vi "输出调用01.vi"(0 "输出簇":cluster{"用户名":string, "项目名称":string}, 7 "数组":string[][](array[string]), 9 "字符串":string, 11 "输出簇 2":T1, 12 "Str引用句柄":refnum<vi>) -> ()   [LabVIEW 2020]
uses:
  <vilib>/numeric/Random Number (Range) DBL.vi
  <vilib>/Utility/miscctls.llb/LVDateTimeRec.ctl
panel:
  out "压力":dbl
  out "数组 6":dbl[][](array[numeric])
  out "水质":dbl
  out "温度":dbl
  out "输出 3":dbl
  out "输出 2":dbl
  out "创建的路径":path
  out "路径 2":path
  out "路径":path
  out "错误输出":errorcluster
  out "数组 5":dbl[](array[numeric])
  out "数组 4":dbl[](array[numeric])
  out "文本":string[](array[string])
  out "数组 3":dbl[](array[numeric])
  out "数组 2":dbl[](array[numeric])
  out "错误输出 2":errorcluster caption="错误输出"
  out "元素":string
  out "数值 3":i32
  out "Numeric":i32
  in  "数值":u32
  out "输出 1":dbl
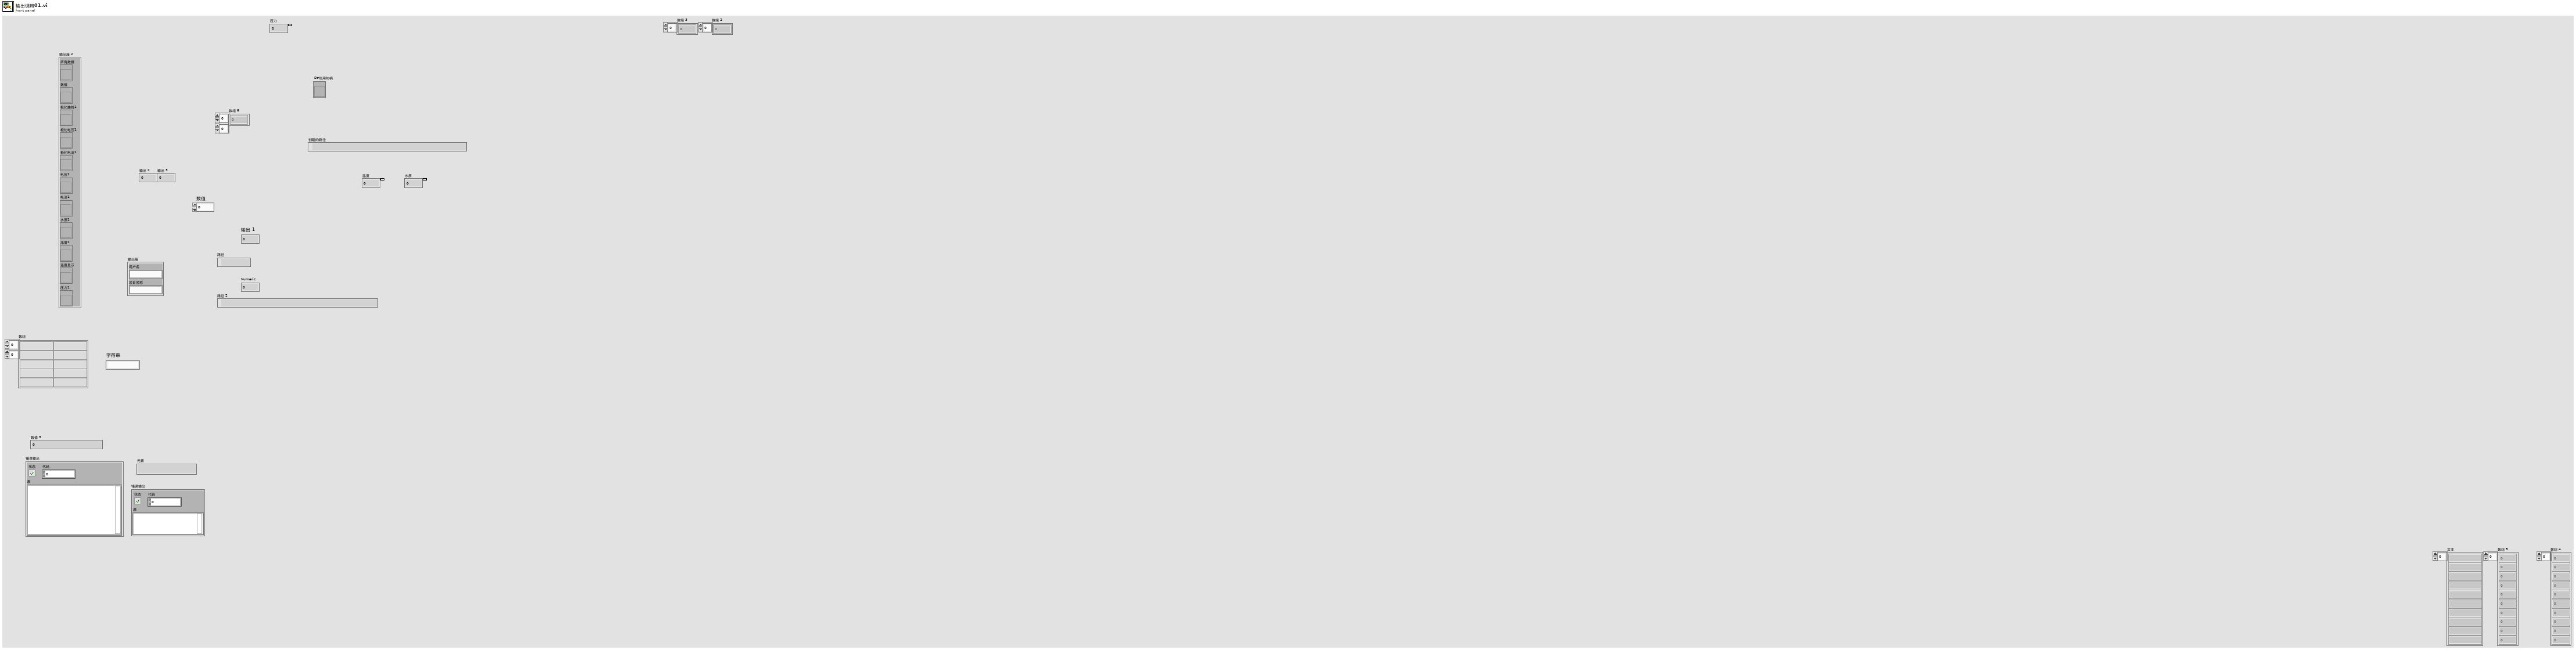
[diagram p1: front panel]
types:
  T1 = cluster{"所有数据":refnum<vi>, "数值":refnum<vi>, "极化曲线1":refnum<vi>, "极化电压1":refnum<vi>, "极化电流1":refnum<vi>, "电压1":refnum<vi>, "电流1":refnum<vi>, "水质1":refnum<vi>, "温度1":refnum<vi>, "温度显示":refnum<vi>, "压力1":refnum<vi>}
  T2 = enum16{"open", "replace", "create", "open or create", "replace or create", "replace or create with confirmation"}
  T3 = typedef "LVDateTimeRec.ctl" = cluster{"fractional second":dbl, "second":i32, "minute":i32, "hour":i32, "day of month":i32, "month":i32, "year":i32, "day of week":i32, "day of year":i32, "DST":i32}
  T4 = enum16{"open", "open or create", "create or replace", "create", "open (read-only)"}
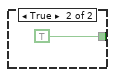
[diagram p3: hidden frame]
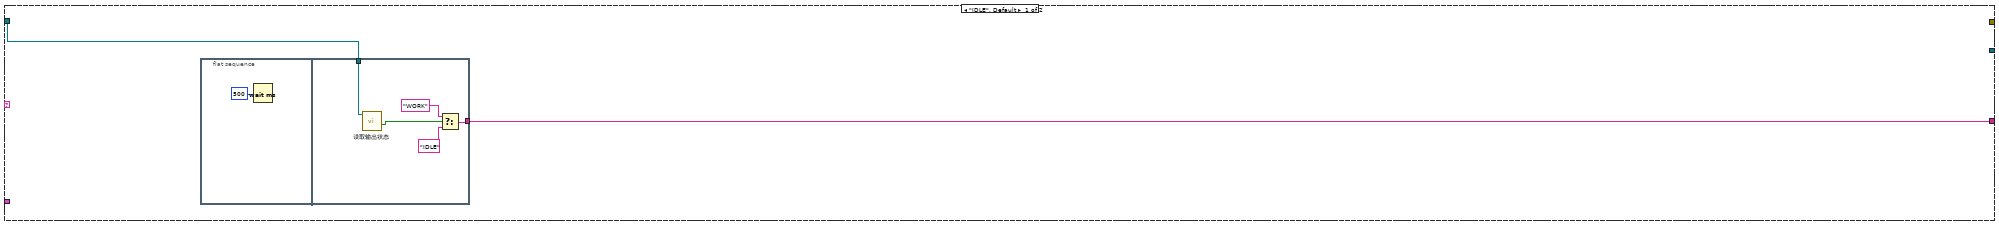
[diagram p5: hidden frame]
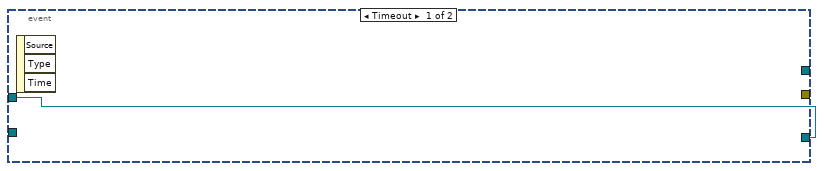
[diagram p6: hidden frame]
diagram:
  w16 = "\\" ("string")
  (unwired) dbl[] [] ("数组 4")
  n1 = Unbundle By Name("输出簇") -> ("用户名"=w13:string, "项目名称"=w12:string)
  n2 = Get Date/Time In Seconds() -> (seconds since 1Jan1904=w34:timestamp)
  n3 = Format Date/Time String(time format string (%c)="%y-%m-%d[%H-%M]", seconds (now)=w34) -> (date/time string=w15:string)  [unwired: 1 in]
  n4 = property on="输出簇 2" class="Clust (严格)"() -> ("Value"=w6:T1)  [unwired: 2 in, 2 out]
  n5 = Concatenate Strings("C:\\Users\\526computer\\Desktop", w16, "TEMPDATA\\" ("string"), w13, w16, w12, w16, "CH1\\" ("string"), w15) -> (w32:string)
  n6 = String To Path(string=w32) -> (path=w31:path)
  n7 = Create Folder(path (use dialog)=w31) -> (created path=w4:path)  [unwired: 2 in, 2 out]
  "创建的路径" <- w4
  n8 = Path To String(path=w4) -> (string=w30:string)
  n9 = Path To String(path=w4) -> (string=w2:string)
  n10 = Concatenate Strings(w30, "\\" ("string"), "通道1 索引.txt" ("string")) -> (w22:string)
  n11 = property class="Str"(reference="Str引用句柄", "Value"=w2) -> ()  [unwired: 1 in, 2 out]
  n12 = String To Path(string=w22) -> (path=w21:path)
  "路径 2" <- w21
  n13 = Unbundle By Name(w6) -> ("极化曲线1"=w11:refnum<vi>)
  n14 = property on="数组 6" class="Arr (严格)"("Value"=dbl[][] [] ("数组 6")) -> (error out=w8:errorcluster)  [unwired: 2 in, 1 out]
  n15 = Open/Create/Replace File(file path (use dialog)=w21, operation (0:open)=T2."replace or create") -> (refnum out=w20:refnum<file>)  [unwired: 4 in, 2 out]
  n16 = while {
    tunnel: w20 -> [w46]
    tunnel: [w45] -> w18
    tunnel: [w44] -> w19
    shift-right: [w42] -> _
    shift-left: w11 -> [w43]
    tunnel: w8 -> [_]
    stop <- FALSE stop-if-true
    n17 = event shown="[1] \"数值\": 值改变" {
      selector: _ -> [_ _]
      dyn-events: _ -> [_ _]
      timeout: 100 -> [_ _]
      tunnel: w46 -> [_ w64]
      tunnel: [_ w58] -> w45
      tunnel: [_ w57] -> w44
      tunnel: w43 -> [w49 w53]
      tunnel: [w49 w52] -> w42
      event Timeout {
        n18 = event-data() -> ()  [unwired: 1 in, 3 out]
      }
      event "数值": Value Change {
        n19 = event-data() -> ()  [unwired: 1 in, 6 out]
        n20 = local read "输出 3"() -> (w54:dbl)
        n21 = local read "输出 2"() -> (w55:dbl)
        n22 = property on="Numeric" class="DigNum (严格)"() -> ("Value"=w63:i32)  [unwired: 2 in, 2 out]
        n23 = Build Array(w55, w54) -> (w56:dbl[])
        n24 = Format Into String(w63) -> (resulting string=w62:string)  [unwired: 3 in, 1 out]
        n25 = property on="数组 6" class="Arr (严格)"() -> ("Value"=w51:dbl[][])  [unwired: 2 in, 2 out]
        n26 = Write to Text File(file (use dialog)=w64, text=w62) -> (refnum out=w61:refnum<file>, error out=w60:errorcluster)  [unwired: 2 in, 1 out]
        n27 = Insert Into Array(array=w51, new element=w56) -> (w50:dbl[][])  [unwired: 2 in]
        n28 = property on="数组 6" class="Arr (严格)"("Value"=w50) -> ()  [unwired: 2 in, 2 out]
        n29 = Write to Text File(file (use dialog)=w61, text="\r\n", error in=w60) -> (refnum out=w58:refnum<file>, error out=w57:errorcluster)  [unwired: 1 in, 1 out]
        n30 = property class="Arr (严格)"(reference=w53, "Value"=w50) -> (reference out=w52:refnum<vi>)  [unwired: 1 in, 1 out]
      }
    }
  }
  n31 = Path To String(path=w4) -> (string=w25:string)
  n32 = Concatenate Strings(w25, "\\" ("string"), "通道1 数据.txt" ("string")) -> (w24:string)
  n33 = String To Path(string=w24) -> (path=w23:path)
  "路径" <- w23
  n34 = Close File(refnum=w18, error in=w19) -> ()  [unwired: 2 out]
  n35 = Open/Create/Replace File(file path (use dialog)=w23, operation (0:open)=T2."replace or create" ("操作(0:open)")) -> (refnum out=w10:refnum<file>, error out=w38:errorcluster)  [unwired: 4 in, 1 out]
  n36 = disable-structure shown="禁用" {
    disable-tunnel: [w65 _] -> w41
    frame Disabled {
      n37 = flat-sequence {
        tunnel: [w89] -> w84
        tunnel: [w86] -> w83
        tunnel: w84 -> [w93]
        tunnel: [w93] -> w82
        tunnel: [w92] -> w81
        tunnel: w83 -> [w92]
        tunnel: ["字符串"] -> w80
        tunnel: w82 -> [w95]
        tunnel: w81 -> [w96]
        tunnel: [w96] -> w79
        tunnel: [w95] -> w78
        tunnel: [w94] -> w77
        tunnel: w80 -> [w94]
        tunnel: w79 -> [w103]
        tunnel: w78 -> [w104]
        tunnel: [w106] -> w76
        tunnel: [w105] -> w75
        tunnel: [w104] -> w74
        tunnel: [w103] -> w73
        tunnel: [w102] -> w65
        tunnel: w77 -> [w101]
        tunnel: w76 -> [w119]
        tunnel: w75 -> [w118]
        tunnel: [w115] -> w72
        tunnel: w74 -> [w115]
        tunnel: [w114] -> w71
        tunnel: w73 -> [w114]
        tunnel: [w109] -> w70
        tunnel: [w108] -> w69
        tunnel: ["输出簇 2"] -> w68
        tunnel: w72 -> [w148]
        tunnel: w71 -> [w152]
        tunnel: w70 -> [w151]
        tunnel: w69 -> [w150]
        tunnel: [w149] -> w67
        tunnel: [w145] -> w66
        tunnel: w68 -> [w144]
        tunnel: w67 -> [w205]
        tunnel: w66 -> [w203]
        frame #0 {
          n38 = property on="数值" class="DigNum (严格)"("Value"=i64 0 ("数值")) -> ()  [unwired: 2 in, 2 out]
          n39 = Index Array(array="数组", index (col)=5 ("禁用的索引 (列)")) -> (element=w86:string[])  [unwired: 1 in]
          n40 = Index Array(array="数组", index (col)=3 ("禁用的索引 (列)")) -> (element=w89:string[])  [unwired: 1 in]
        }
        frame #1 {
          n41 = VISA Close(VISA resource name="字符串") -> ()  [unwired: 1 in, 1 out]
        }
        frame #2 {
        }
        frame #3 {
          n42 = VISA Open(VISA resource name=w101) -> (VISA resource name=w102:refnum<visa-resource-name>, error out=w99:errorcluster)  [unwired: 4 in]
          n43 = call "remote.vi"("error in (no error)"=w99, "VISA resource name"=w102) -> ("error out"=w97:errorcluster, "VISA resource name out"=w98:refnum<visa-resource-name>)  [unwired: 8 in]
          n44 = call "enableoutput.vi"("error in (no error)"=w97, "Enable OutPut(True)"=FALSE, "VISA resource name"=w98) -> ("error out"=w105:errorcluster, "VISA resource name out"=w106:refnum<visa-resource-name>)  [unwired: 7 in]
        }
        frame #4 {
          n45 = flat-sequence {
            tunnel: w119 -> [w124]
            tunnel: w118 -> [w123]
            tunnel: [w121] -> w117
            tunnel: [w120] -> w116
            tunnel: w117 -> [w130]
            tunnel: w116 -> [w129]
            tunnel: [w126] -> w113
            tunnel: [w125] -> w112
            tunnel: w113 -> [w136]
            tunnel: w112 -> [w135]
            tunnel: [w133] -> w111
            tunnel: [w132] -> w110
            tunnel: w111 -> [w142]
            tunnel: w110 -> [w141]
            tunnel: [w138] -> w109
            tunnel: [w137] -> w108
            frame #0 {
              n46 = call "priority.vi"("error in (no error)"=w123, "字符串"="CURR", "VISA resource name"=w124) -> ("error out"=w120:errorcluster, "VISA resource name out"=w121:refnum<visa-resource-name>)  [unwired: 7 in]
            }
            frame #1 {
              n47 = call "初始化电压电流.vi"("error in (no error)"=w129, "输入 2"=0.1, "输入 1"=15.0, "VISA resource name"=w130) -> ("error out"=w125:errorcluster, "VISA resource name out"=w126:refnum<visa-resource-name>)  [unwired: 6 in]
            }
            frame #2 {
              n48 = call "限制电流.vi"("error in (no error)"=w135, "OCP Delay(0)"=3.0, "数值"=120.0 ("OCP Level(0)"), "VISA resource name"=w136) -> ("error out"=w132:errorcluster, "VISA resource name out"=w133:refnum<visa-resource-name>)  [unwired: 6 in]
            }
            frame #3 {
              n49 = call "限制电压.vi"("error in (no error)"=w141, "OVP Delay(0)"=3.0, "OVP Level(0)"=20.0, "VISA resource name"=w142) -> ("error out"=w137:errorcluster, "VISA resource name out"=w138:refnum<visa-resource-name>)  [unwired: 6 in]
            }
          }
        }
        frame #5 {
          n50 = Unbundle By Name(w144) -> ("数值"=w143:refnum<vi>)
          n51 = Search 1D Array(1D array=w148, element=" " ("元素")) -> (index of element=w146:i32)  [unwired: 1 in]
          n52 = for {
            N: w146 -> [_]
            tunnel: w152 -> [w174] mode=indexing
            tunnel: w148 -> [w171] mode=indexing
            tunnel: w150 -> [w169]
            shift-right: [w164] -> w149
            shift-left: w151 -> [w170]
            tunnel: [w161] -> w145
            shift-right: [w155] -> _
            shift-left: w143 -> [w156]
            i -> [w154]
            n53 = Scan From String(input string=w174) -> (output 1=w173:dbl)  [unwired: 4 in, 3 out]
            n54 = Scan From String(input string=w171) -> (output 1=w168:dbl)  [unwired: 4 in, 3 out]
            "输出 1" <- w168
            n55 = Multiply(x=w173, y=1000.0) -> (x*y=w165:dbl)
            n56 = flat-sequence {
              tunnel: w170 -> [w179]
              tunnel: w169 -> [w178]
              tunnel: w168 -> [w177]
              tunnel: [w176] -> w167
              tunnel: [w175] -> w166
              tunnel: w167 -> [w182]
              tunnel: w166 -> [w183]
              tunnel: [w181] -> w163
              tunnel: [w180] -> w162
              tunnel: w165 -> [w193]
              tunnel: w163 -> [w192]
              tunnel: [w192] -> w160
              tunnel: [w191] -> w158
              tunnel: w162 -> [w191]
              tunnel: w160 -> [w198]
              tunnel: [w198] -> w159
              tunnel: w158 -> [w197]
              tunnel: [w197] -> w157
              tunnel: w156 -> [w196]
              tunnel: [w195] -> w155
              tunnel: w153 -> [w194]
              tunnel: [w201] -> w164
              tunnel: w159 -> [w202]
              tunnel: w157 -> [w200]
              tunnel: [w199] -> w161
              frame #0 {
                n57 = call "设置电流.vi"("error in (no error)"=w178, "输入 1"=w177, "VISA resource name"=w179) -> ("error out"=w175:errorcluster, "VISA resource name out"=w176:refnum<visa-resource-name>)  [unwired: 7 in]
              }
              frame #1 {
                n58 = First Call?() -> (First Call?: T/F=w184:bool)
                n59 = case shown="真" w184 {
                  tunnel: w182 -> [w185 w190]
                  tunnel: w183 -> [_ w189]
                  tunnel: [w185 w187] -> w181
                  tunnel: [_ w186] -> w180
                  frame False {
                  }
                  frame True {
                    n60 = call "enableoutput.vi"("error in (no error)"=w189, "Enable OutPut(True)"=TRUE, "VISA resource name"=w190) -> ("error out"=w186:errorcluster, "VISA resource name out"=w187:refnum<visa-resource-name>)  [unwired: 7 in]
                  }
                }
              }
              frame #2 {
                n61 = Wait (ms)(milliseconds to wait=w193) -> ()  [unwired: 1 out]
              }
              frame #3 {
                n62 = property on="数值" class="DigNum (严格)"("Val(Sgnl)"=w194) -> ()  [unwired: 2 in, 2 out]
                n63 = property class="DigNum (严格)"(reference=w196, "Val(Sgnl)"=w194) -> (reference out=w195:refnum<vi>)  [unwired: 1 in, 1 out]
              }
              frame #4 {
                n64 = call "remote.vi"("error in (no error)"=w200, "VISA resource name"=w202) -> ("error out"=w199:errorcluster, "VISA resource name out"=w201:refnum<visa-resource-name>)  [unwired: 8 in]
              }
            }
            n65 = Increment(x=w154) -> (x+1=w153:i32)
          }
        }
        frame #6 {
          n66 = flat-sequence {
            tunnel: w205 -> [w209]
            tunnel: [w208] -> w204
            tunnel: w203 -> [w206]
            tunnel: w204 -> [w210]
            frame #0 {
              n67 = call "enableoutput.vi"("error in (no error)"=w206, "Enable OutPut(True)"=FALSE, "VISA resource name"=w209) -> ("VISA resource name out"=w208:refnum<visa-resource-name>)  [unwired: 7 in, 1 out]
            }
            frame #1 {
              n68 = VISA Close(VISA resource name=w210) -> ()  [unwired: 1 in, 1 out]
            }
            frame #2 {
              n69 = flat-sequence {
                tunnel: [w230] -> w223
                tunnel: [w229] -> w222
                tunnel: [w228] -> w221
                tunnel: [w227] -> w220
                tunnel: [w226] -> w219
                tunnel: [w224] -> w212
                tunnel: w223 -> [w279]
                tunnel: w222 -> [w278]
                tunnel: [w296] -> w213
                tunnel: [w295] -> w214
                tunnel: w221 -> [w291]
                tunnel: [w290] -> w215
                tunnel: w220 -> [w282]
                tunnel: w219 -> [w283]
                tunnel: [w280] -> w216
                tunnel: [w281] -> w217
                tunnel: [w280] -> w218
                tunnel: w212 -> [w274]
                tunnel: [w273] -> w211
                tunnel: w218 -> [w354]
                tunnel: w217 -> [w353]
                tunnel: w216 -> [w372]
                tunnel: w215 -> [w378]
                tunnel: w214 -> [w386]
                tunnel: w213 -> [w385]
                tunnel: w211 -> [w303]
                frame #0 {
                  n70 = property on="路径" class="Path"() -> ("Value"=w225:path)  [unwired: 2 in, 2 out]
                  n71 = Open/Create/Replace File(file path (use dialog)=w225, operation (0:open)=T2."open" ("操作(0:open)")) -> (refnum out=w233:refnum<file>, error out=w232:errorcluster)  [unwired: 4 in, 1 out]
                  n72 = while {
                    tunnel: w233 -> [w270]
                    tunnel: w232 -> [w268]
                    tunnel: [w267] -> w231
                    tunnel: [w241] -> w230 mode=indexing
                    tunnel: [w240] -> w229 mode=indexing
                    tunnel: [w256] -> _
                    tunnel: [w244] -> w228 mode=indexing
                    tunnel: [w239] -> w227 mode=indexing
                    tunnel: [w238] -> w226 mode=indexing
                    tunnel: [w235] -> w224 mode=indexing
                    i -> [w237]
                    stop <- w257 stop-if-true
                    n73 = Read from Text File(file (use dialog)=w270, count=1 ("计数"), error in=w268) -> (refnum out=w267:refnum<file>, text=w261:string[], error out=w256:errorcluster)  [unwired: 1 in, 1 out]
                    n74 = Unbundle By Name(w256) -> ("status"=w264:bool, "code"=w266:i32)
                    n75 = Equal?(x=w266, y=4) -> (x = y?=w263:bool)
                    n76 = Index Array(array=w261, index=0 ("索引")) -> (element=w258:string)
                    "元素" <- w258
                    n77 = And(x=w264, y=w263) -> (x .and. y?=w262:bool)
                    n78 = case shown="假" w262 {
                      tunnel: [FALSE TRUE] -> w257
                      frame False {
                      }
                      frame True {
                      }
                    }
                    n79 = Search/Split String(string=w258, search string/char (-)="电流：" ("正则表达式")) -> (substring before match=w253:string, match + rest of string=w243:string)  [unwired: 1 in, 1 out]
                    n80 = Scan From String(format string="%d-%d-%d %d:%d:%d" ("格式字符串"), input string=w253) -> (error out=→"错误输出 2":errorcluster, output 1=w252:i32, output 2=w251:i32, output 3=w250:i32, output 4=w249:i32, output 5=w248:i32, output 6=w247:i32)  [unwired: 8 in, 2 out]
                    n81 = Bundle By Name(cluster=T3 {"fractional second"=0.9035696983337402, "second"=34, "minute"=35, "hour"=15, "day of month"=21, "month"=2, "year"=2022, "day of week"=2, "day of year"=52, "DST"=0} ("日期时间记录"), "second"=w247, "minute"=w248, "hour"=w249, "day of month"=w250, "month"=w251, "year"=w252) -> (w245:T3)
                    n82 = Scan From String(format string="电流：%f 电压：%f 温度：%f 水质：%f 压力：%f" ("格式字符串"), input string=w243) -> (error out=w236:errorcluster, output 1=w241:dbl, output 2=w240:dbl, output 3=w239:dbl, output 4=w238:dbl, output 5=w235:dbl)  [unwired: 7 in, 2 out]
                    n83 = call <vilib>:"Clear Errors.vi"("error in (no error)"=w236) -> ()  [unwired: 5 in, 2 out]
                    n84 = Date/Time To Seconds(2:w245) -> (0:w244:timestamp)  [unwired: 1 in]
                    "数值 3" <- w237
                  }
                  n85 = Close File(refnum=w231) -> ()  [unwired: 1 in, 2 out]
                }
                frame #1 {
                  n86 = Array Size(array=w278) -> (size(s)=w298:i32)
                  n87 = Array Size(array=w279) -> (size(s)=w301:i32)
                  n88 = Array Size(array=w291) -> (size(s)=w293:i32)
                  n89 = Array Size(array=w274) -> (size(s)=w275:i32)
                  n90 = Decrement(x=w298) -> (x-1=w299:i32)
                  n91 = Decrement(x=w301) -> (x-1=w300:i32)
                  n92 = Decrement(x=w293) -> (x-1=w294:i32)
                  n93 = Array Size(array=w282) -> (size(s)=w289:i32)
                  n94 = Array Size(array=w283) -> (size(s)=w288:i32)
                  n95 = Decrement(x=w275) -> (x-1=w277:i32)
                  n96 = Decrement(x=w289) -> (x-1=w287:i32)
                  n97 = Decrement(x=w288) -> (x-1=w284:i32)
                  n98 = Delete From Array(array=w274, length=1 ("长度"), index=w277) -> (array with subset deleted=w273:dbl[])  [unwired: 1 out]
                  n99 = Delete From Array(array=w282, length=1 ("长度"), index=w287) -> (array with subset deleted=w280:dbl[])  [unwired: 1 out]
                  n100 = Delete From Array(array=w278, length=1 ("长度"), index=w299) -> (array with subset deleted=w295:dbl[])  [unwired: 1 out]
                  n101 = Delete From Array(array=w279, length=1 ("长度"), index=w300) -> (array with subset deleted=w296:dbl[])  [unwired: 1 out]
                  n102 = Delete From Array(array=w291, length=1 ("长度"), index=w294) -> (array with subset deleted=w290:timestamp[])  [unwired: 1 out]
                  n103 = Delete From Array(array=w283, length=1 ("长度"), index=w284) -> (array with subset deleted=w281:dbl[])  [unwired: 1 out]
                  "数组 3" <- w279
                  "数组 2" <- w278
                }
                frame #2 {
                  w340 = "极化" ("组名称输入（无标题）")
                  w319 = "数据" ("组名称")
                  n104 = property on="创建的路径" class="Path"() -> ("Value"=w322:path)  [unwired: 2 in, 2 out]
                  n105 = Array Max & Min(array=w303) -> (max value=w305:dbl, max index (indices)=w307:i32, min value=w306:dbl, min index (indices)=w308:i32)
                  n106 = Array Max & Min(array=w372) -> (max value=w347:dbl, max index (indices)=w345:i32, min value=w346:dbl, min index (indices)=w344:i32)
                  n107 = Array Max & Min(array=w353) -> (max value=w351:dbl, max index (indices)=w349:i32, min value=w350:dbl, min index (indices)=w348:i32)
                  n108 = Array Size(array=w378) -> (size(s)=w377:i32)
                  n109 = Array Max & Min(array=w386) -> (max value=w399:dbl, max index (indices)=w394:i32, min value=w398:dbl, min index (indices)=w393:i32)
                  n110 = Array Max & Min(array=w385) -> (max value=w401:dbl, max index (indices)=w395:i32, min value=w402:dbl, min index (indices)=w396:i32)
                  n111 = Index Array(array=w378, index=0 ("索引")) -> (element=w375:timestamp)
                  n112 = Build Array(w306, w305, w307, w308) -> (w304:dbl[])
                  n113 = Build Array(w351, w350, w349, w348) -> (w362:dbl[])
                  n114 = Build Array(w347, w346, w345, w344) -> (w363:dbl[])
                  n115 = Decrement(x=w377) -> (x-1=w376:i32)
                  n116 = Build Array(w398, w399, w394, w393) -> (w397:dbl[])
                  n117 = Build Array(w402, w401, w396, w395) -> (w400:dbl[])
                  n118 = Path To String(path=w322) -> (string=w323:string)
                  n119 = Index Array(array=w378, index=w376) -> (element=w374:timestamp)
                  n120 = Get Date/Time In Seconds() -> (seconds since 1Jan1904=w418:timestamp)
                  n121 = Format Date/Time String(time format string (%c)="%Y-%m-%d-%H-%M-%S" ("时间格式字符串(%c)"), seconds (now)=w418) -> (date/time string=w325:string)  [unwired: 1 in]
                  n122 = Concatenate Strings(w323, "\\" ("字符串"), w325, ".tdms" ("字符串")) -> (w419:string)
                  n123 = String To Path(string=w419) -> (path=w420:path)
                  n124 = Build Array(w375, w374) -> (w373:timestamp[])
                  n125 = TDMS Open(5:FALSE ("创建索引文件？(T)"), 10:T4."create or replace" ("操作(0:open)"), 11:w420) -> (0:w331:errorcluster, 3:w333:refnum<k34>)  [unwired: 4 in]
                  n126 = Build Array("电解水实验" ("组名称"), "孙成，王彪" ("组名称"), w325, "极化曲线" ("组名称")) -> (w324:string[])
                  n127 = TDMS Set Properties(5:w324, 7:string[] ["Title", "Author", "Date/Time", "type"] ("属性名称"), 8:w331, 11:w333) -> (0:w330:errorcluster, 3:w332:refnum<k34>)  [unwired: 2 in, 2 out]
                  n128 = TDMS Set Properties(5:w373, 7:string[] ["最小值", "最大值"] ("属性名称"), 8:w330, 9:"测试时间" ("通道名称"), 10:w319, 11:w332) -> (0:w409:errorcluster, 3:w410:refnum<k34>)  [unwired: 2 out]
                  n129 = TDMS Set Properties(5:w400, 7:string[] ["最小值", "最大值", "最小索引", "最大索引"] ("属性名称"), 8:w409, 9:"电流" ("通道名称"), 10:w319, 11:w410) -> (0:w403:errorcluster, 3:w406:refnum<k34>)  [unwired: 2 out]
                  n130 = TDMS Set Properties(5:w397, 7:string[] ["最小值", "最大值", "最小索引", "最大索引"] ("属性名称"), 8:w403, 9:"电压" ("通道名称"), 10:w319, 11:w406) -> (0:w366:errorcluster, 3:w367:refnum<k34>)  [unwired: 2 out]
                  n131 = TDMS Set Properties(5:w363, 7:string[] ["最小值", "最大值", "最小索引", "最大索引"] ("属性名称"), 8:w366, 9:"温度" ("通道名称"), 10:w319, 11:w367) -> (0:w364:errorcluster, 3:w365:refnum<k34>)  [unwired: 2 out]
                  n132 = TDMS Set Properties(5:w362, 7:string[] ["最小值", "最大值", "最小索引", "最大索引"] ("属性名称"), 8:w364, 9:"水质" ("通道名称"), 10:w319, 11:w365) -> (0:w316:errorcluster, 3:w318:refnum<k34>)  [unwired: 2 out]
                  n133 = TDMS Set Properties(5:w304, 7:string[] ["最小值", "最大值", "最小索引", "最大索引"] ("属性名称"), 8:w316, 9:"压力" ("通道名称"), 10:w319, 11:w318) -> (0:w315:errorcluster, 3:w317:refnum<k34>)  [unwired: 2 out]
                  n134 = TDMS Write(0:w317, 5:"数据" ("组名称输入（无标题）"), 7:string[] ["电流"] ("通道名输入（无标题）"), 9:w385, 11:w315) -> (4:w389:refnum<k34>, 15:w388:errorcluster)  [unwired: 1 in, 2 out]
                  n135 = TDMS Write(0:w389, 5:"数据" ("组名称输入（无标题）"), 7:string[] ["电压"] ("通道名输入（无标题）"), 9:w386, 11:w388) -> (4:w381:refnum<k34>, 15:w380:errorcluster)  [unwired: 1 in, 2 out]
                  n136 = TDMS Write(0:w381, 5:"数据" ("组名称输入（无标题）"), 7:string[] ["测试时间"] ("通道名输入（无标题）"), 9:w378, 11:w380) -> (4:w356:refnum<k34>, 15:w355:errorcluster)  [unwired: 1 in, 2 out]
                  n137 = flat-sequence {
                    tunnel: [w422] -> w343
                    tunnel: w343 -> [w429]
                    tunnel: [w428] -> w335
                    tunnel: [w427] -> w334
                    frame #0 {
                      n138 = property on="路径 2" class="Path"() -> ("Value"=w421:path)  [unwired: 2 in, 2 out]
                      n139 = Open/Create/Replace File(file path (use dialog)=w421, operation (0:open)=T2."open" ("操作(0:open)")) -> (refnum out=w426:refnum<file>)  [unwired: 4 in, 2 out]
                      n140 = Read from Text File(file (use dialog)=w426, count=-1 ("计数")) -> (refnum out=w423:refnum<file>, text=w422:string[])  [unwired: 2 in, 2 out]
                      "文本" <- w422
                      n141 = Close File(refnum=w423) -> ()  [unwired: 1 in, 2 out]
                    }
                    frame #1 {
                      n142 = for {
                        tunnel: w429 -> [w438] mode=indexing
                        tunnel: [w436] -> w428 mode=indexing
                        tunnel: [w435] -> w427 mode=indexing
                        n143 = Scan From String(format string="%d" ("格式字符串"), input string=w438) -> (output 1=w434:i32)  [unwired: 3 in, 3 out]
                        n144 = property on="数组 3" class="Arr (严格)"() -> ("Value"=w430:dbl[])  [unwired: 2 in, 2 out]
                        n145 = Decrement(x=w434) -> (x-1=w433:i32)
                        n146 = Decrement(x=w434) -> (x-1=w432:i32)
                        n147 = Index Array(array=w430, index=w433) -> (element=w436:dbl)
                        n148 = property on="数组 2" class="Arr (严格)"() -> ("Value"=w431:dbl[])  [unwired: 2 in, 2 out]
                        n149 = Index Array(array=w431, index=w432) -> (element=w435:dbl)
                      }
                      "数组 5" <- w428
                      "数组 4" <- w427
                    }
                  }
                  n150 = TDMS Write(0:w356, 5:"数据" ("组名称输入（无标题）"), 7:string[] ["温度"] ("通道名输入（无标题）"), 9:w354, 11:w355) -> (4:w352:refnum<k34>, 15:w361:errorcluster)  [unwired: 1 in, 2 out]
                  n151 = TDMS Write(0:w352, 5:"数据" ("组名称输入（无标题）"), 7:string[] ["水质"] ("通道名输入（无标题）"), 9:w353, 11:w361) -> (4:w312:refnum<k34>, 15:w310:errorcluster)  [unwired: 1 in, 2 out]
                  n152 = TDMS Write(0:w312, 5:"数据" ("组名称输入（无标题）"), 7:string[] ["压力"] ("通道名输入（无标题）"), 9:w303, 11:w310) -> (4:w311:refnum<k34>, 15:w309:errorcluster)  [unwired: 1 in, 2 out]
                  n153 = TDMS Write(0:w311, 5:w340, 7:string[] ["电流"] ("通道名输入（无标题）"), 9:w335, 11:w309) -> (4:w342:refnum<k34>, 15:w341:errorcluster)  [unwired: 1 in, 2 out]
                  n154 = TDMS Write(0:w342, 5:w340, 7:string[] ["电压"] ("通道名输入（无标题）"), 9:w334, 11:w341) -> (4:w337:refnum<k34>, 15:w336:errorcluster)  [unwired: 1 in, 2 out]
                  n155 = TDMS Close(8:w336, 11:w337) -> (0:→"错误输出":errorcluster)  [unwired: 1 out]
                }
              }
            }
            frame #3 {
              n156 = Request Deallocation(TRUE ("标志")) -> ()
            }
            frame #4 {
              n157 = Stop(stop? (T)=TRUE ("停止？(T)")) -> ()
            }
          }
        }
      }
    }
    frame Enabled {
    }
  }
  n158 = property on="输出簇 2" class="Clust (严格)"() -> ("Value"=w7:T1)  [unwired: 2 in, 2 out]
  n159 = while {
    shift-right: [w444] -> _
    shift-left: "IDLE" -> [w450]
    tunnel: w41 -> [w449]
    tunnel: w10 -> [w448]
    tunnel: w38 -> [w447]
    tunnel: [w446] -> w37
    tunnel: [w445] -> w36
    tunnel: w7 -> [w441]
    i -> [w443]
    stop <- FALSE stop-if-true
    n160 = Wait (ms)(milliseconds to wait=u32 500 ("等待时间（毫秒）")) -> ()  [unwired: 1 out]
    n161 = case shown="\"WORK\"" w450 {
      tunnel: [w453 w506] -> w444
      tunnel: w449 -> [w452 w514]
      tunnel: w448 -> [_ w513]
      tunnel: w447 -> [_ w511]
      tunnel: [_ w508] -> w446
      tunnel: [_ w507] -> w445
      tunnel: w441 -> [_ w493]
      frame "IDLE", Default {
        n162 = flat-sequence {
          tunnel: [w456] -> w453
          tunnel: w452 -> [w455]
          frame #0 {
            n163 = Wait (ms)(milliseconds to wait=u32 500 ("等待时间（毫秒）")) -> ()  [unwired: 1 out]
          }
          frame #1 {
            n164 = call "读取输出状态.vi"("VISA resource name"=w455) -> ("x = y?"=w459:bool)  [unwired: 7 in, 3 out]
            n165 = Select(t="WORK", s=w459, f="IDLE") -> (s? t:f=w456:string)
          }
        }
      }
      frame "WORK" {
        n166 = Unbundle By Name(w493) -> ("所有数据"=w471:refnum<vi>, "极化电压1"=w469:refnum<vi>, "极化电流1"=w492:refnum<vi>, "电压1"=w491:refnum<vi>, "电流1"=w490:refnum<vi>, "水质1"=w470:refnum<vi>, "温度1"=w468:refnum<vi>, "压力1"=w463:refnum<vi>)  [unwired: 3 out]
        n167 = flat-sequence {
          tunnel: [w526] -> w517
          tunnel: [w525] -> w516
          tunnel: w514 -> [w524]
          tunnel: w513 -> [w522]
          tunnel: [w523] -> w512
          tunnel: w511 -> [w523]
          tunnel: [w522] -> w510
          tunnel: [w518] -> w509
          tunnel: w492 -> [w521]
          tunnel: [w518] -> w486
          tunnel: [w518] -> w460
          tunnel: w517 -> [w538]
          tunnel: w516 -> [w537]
          tunnel: [w535] -> w505
          tunnel: [w534] -> w503
          tunnel: w512 -> [w532]
          tunnel: w510 -> [w533]
          tunnel: [w533] -> w501
          tunnel: [w532] -> w499
          tunnel: [w531] -> w497
          tunnel: w509 -> [w531]
          tunnel: [w528] -> w495
          tunnel: [w528] -> w489
          tunnel: [w530] -> w487
          tunnel: w486 -> [w530]
          tunnel: [w528] -> w484
          tunnel: w469 -> [w529]
          tunnel: w460 -> [w528]
          tunnel: w505 -> [w555]
          tunnel: [w555] -> w504
          tunnel: w503 -> [w554]
          tunnel: [w554] -> w502
          tunnel: w501 -> [w553]
          tunnel: [w553] -> w500
          tunnel: w499 -> [w552]
          tunnel: [w552] -> w498
          tunnel: w497 -> [w551]
          tunnel: [w551] -> w496
          tunnel: w495 -> [w550]
          tunnel: [w550] -> w494
          tunnel: w491 -> [w549]
          tunnel: w490 -> [w541]
          tunnel: w489 -> [w546]
          tunnel: [w540] -> w488
          tunnel: w487 -> [w540]
          tunnel: [w539] -> w485
          tunnel: w484 -> [w539]
          tunnel: [w643] -> w483
          tunnel: w504 -> [w643]
          tunnel: w502 -> [w626]
          tunnel: w500 -> [w630]
          tunnel: w498 -> [w629]
          tunnel: w496 -> [w628]
          tunnel: w494 -> [w616]
          tunnel: [w627] -> w481
          tunnel: [w626] -> w479
          tunnel: [w625] -> w507
          tunnel: [w612] -> w477
          tunnel: w488 -> [w612]
          tunnel: [w611] -> w475
          tunnel: w485 -> [w611]
          tunnel: [w604] -> w473
          tunnel: w470 -> [w603]
          tunnel: w468 -> [w584]
          tunnel: [w583] -> w466
          tunnel: [w582] -> w464
          tunnel: w463 -> [w568]
          tunnel: [w567] -> w461
          tunnel: w483 -> [w652]
          tunnel: [w652] -> w482
          tunnel: w481 -> [w651]
          tunnel: [w651] -> w480
          tunnel: w479 -> [w650]
          tunnel: [w650] -> w478
          tunnel: w477 -> [w649]
          tunnel: [w649] -> w476
          tunnel: w475 -> [w648]
          tunnel: [w648] -> w474
          tunnel: w473 -> [w647]
          tunnel: [w647] -> w472
          tunnel: [w646] -> w467
          tunnel: w466 -> [w646]
          tunnel: [w645] -> w465
          tunnel: w464 -> [w645]
          tunnel: [w644] -> w462
          tunnel: w461 -> [w644]
          tunnel: [w674] -> w515
          tunnel: w482 -> [w674]
          tunnel: w480 -> [w673]
          tunnel: w478 -> [w672]
          tunnel: [w671] -> w508
          tunnel: w476 -> [w666]
          tunnel: w474 -> [w663]
          tunnel: w472 -> [w657]
          tunnel: w471 -> [w656]
          tunnel: w467 -> [w655]
          tunnel: w465 -> [w654]
          tunnel: w462 -> [w653]
          tunnel: w515 -> [w679]
          tunnel: [w675] -> w506
          frame #0 {
            w527 = 0 items=["Current", "Power", "Voltage", "Capacity", "Temperature", "Time"] ("Fetch Type")
            n168 = call-poly <vilib>:"Random Number (Range).vi"("lower bound (0)"=10.0, "upper bound (100)"=30.0) -> ("number"=w518:dbl)  [unwired: 9 in]
            "输出 2" <- w518
            n169 = call "fetch.vi"("Fetch Type"=w527, "VISA resource name"=w524) -> ("error out"=w525:errorcluster, "VISA resource name out"=w526:refnum<visa-resource-name>)  [unwired: 7 in, 1 out]
            n170 = property class="DigNum (严格)"(reference=w521, "Value"=w518) -> ()  [unwired: 1 in, 2 out]
          }
          frame #1 {
            w536 = 2 items=["Current", "Power", "Voltage", "Capacity", "Temperature", "Time"] ("Fetch Type")
            n171 = property class="DigNum (严格)"(reference=w529, "Value"=w528) -> ()  [unwired: 1 in, 2 out]
            n172 = call "fetch.vi"("error in (no error)"=w537, "Fetch Type"=w536, "VISA resource name"=w538) -> ("error out"=w534:errorcluster, "VISA resource name out"=w535:refnum<visa-resource-name>)  [unwired: 6 in, 1 out]
            "输出 3" <- w528
          }
          frame #2 {
            n173 = property class="Arr (严格)"(reference=w549) -> (reference out=w548:refnum<vi>, "Value"=w547:dbl[])  [unwired: 1 in, 1 out]
            n174 = Insert Into Array(array=w547, new element=w546) -> (w545:dbl[])  [unwired: 1 in]
            n175 = property class="Arr (严格)"(reference=w541) -> (reference out=w542:refnum<vi>, "Value"=w543:dbl[])  [unwired: 1 in, 1 out]
            n176 = property class="Arr (严格)"(reference=w548, "Value"=w545) -> ()  [unwired: 1 in, 2 out]
            n177 = Insert Into Array(array=w543, new element=w540) -> (w544:dbl[])  [unwired: 1 in]
            n178 = property class="Arr (严格)"(reference=w542, "Value"=w544) -> ()  [unwired: 1 in, 2 out]
          }
          frame #3 {
            (unwired) "时间：" ("字符串")
            n179 = Get Date/Time String() -> (date string=w590:string, time string=w588:string)  [unwired: 3 in]
            n180 = Get Date/Time String() -> (date string=w608:string, time string=w610:string)  [unwired: 3 in]
            n181 = call <vilib>:"Space Constant.vi"() -> ("String"=w602:string)
            n182 = Get Date/Time In Seconds() -> (seconds since 1Jan1904=w642:timestamp)
            n183 = Format Into String(w628) -> (resulting string=w639:string)  [unwired: 3 in, 1 out]
            n184 = Get Date/Time String() -> (date string=w573:string, time string=w575:string)  [unwired: 3 in]
            n185 = Concatenate Strings(w590, "  " ("字符串"), w588) -> (w594:string)
            n186 = Concatenate Strings(w602, "电流：" ("字符串"), w639) -> (w638:string)
            n187 = Concatenate Strings(w608, "  " ("字符串"), w610) -> (w604:string)
            n188 = call-poly <vilib>:"Random Number (Range).vi"("lower bound (0)"=10.0, "upper bound (100)"=30.0) -> ("number"=w556:dbl)  [unwired: 9 in]
            n189 = Format Into String(format string="%.2f" ("格式字符串"), w556) -> (resulting string=w582:string)  [unwired: 2 in, 1 out]
            n190 = Format Into String(format string="%.2f" ("格式字符串"), w556) -> (resulting string=w583:string)  [unwired: 2 in, 1 out]
            n191 = Format Date/Time String(time format string (%c)="%Y-%m-%d %H:%M:%S" ("时间格式字符串(%c)"), seconds (now)=w642) -> (date/time string=w640:string)  [unwired: 1 in]
            n192 = Write to Text File(file (use dialog)=w630, text=w640, error in=w629) -> (refnum out=w637:refnum<file>, error out=w636:errorcluster)  [unwired: 1 in, 1 out]
            n193 = Write to Text File(file (use dialog)=w637, text=w638, error in=w636) -> (refnum out=w633:refnum<file>, error out=w632:errorcluster)  [unwired: 1 in, 1 out]
            n194 = Concatenate Strings(w573, "  " ("字符串"), w575) -> (w569:string)
            n195 = Format Into String(format string="%.2f" ("格式字符串"), w556) -> (resulting string=w567:string)  [unwired: 2 in, 1 out]
            n196 = call <vilib>:"Space Constant.vi"() -> ("String"=w601:string)
            n197 = Format Into String(w616) -> (resulting string=w634:string)  [unwired: 3 in, 1 out]
            n198 = property on="温度" class="DigNum (严格)" props=["Value"]() -> ()  [unwired: 2 in, 3 out]
            n199 = Concatenate Strings(w582, "°C" ("字符串")) -> (w592:string)
            n200 = Concatenate Strings(w583, "MΩ*cm" ("字符串")) -> (w606:string)
            n201 = Concatenate Strings(w567, "bar" ("字符串")) -> (w571:string)
            n202 = property class="Arr (严格)"(reference=w584) -> (reference out=w585:refnum<vi>, "Value"=w587:string[][])  [unwired: 1 in, 1 out]
            n203 = property class="Arr (严格)"(reference=w603) -> (reference out=w615:refnum<vi>, "Value"=w613:string[][])  [unwired: 1 in, 1 out]
            n204 = Concatenate Strings(w601, "电压：" ("字符串"), w634) -> (w635:string)
            n205 = Write to Text File(file (use dialog)=w633, text=w635, error in=w632) -> (refnum out=w620:refnum<file>, error out=w619:errorcluster)  [unwired: 1 in, 1 out]
            n206 = Build Array(w594, w592) -> (w593:string[])
            n207 = Build Array(w604, w606) -> (w605:string[])
            n208 = property class="Arr (严格)"(reference=w568) -> (reference out=w578:refnum<vi>, "Value"=w576:string[][])  [unwired: 1 in, 1 out]
            n209 = call <vilib>:"Space Constant.vi"() -> ("String"=w600:string)
            n210 = Format Into String(w556) -> (resulting string=w624:string)  [unwired: 3 in, 1 out]
            n211 = property on="水质" class="DigNum (严格)" props=["Value"]() -> ()  [unwired: 2 in, 3 out]
            n212 = Build Array(w569, w571) -> (w570:string[])
            n213 = Insert Into Array(array=w587, new element=w593) -> (w586:string[][])  [unwired: 2 in]
            n214 = Insert Into Array(array=w613, new element=w605) -> (w614:string[][])  [unwired: 2 in]
            n215 = Concatenate Strings(w600, "温度：" ("字符串"), w624) -> (w623:string)
            n216 = Write to Text File(file (use dialog)=w620, text=w623, error in=w619) -> (refnum out=w618:refnum<file>, error out=w617:errorcluster)  [unwired: 1 in, 1 out]
            n217 = Insert Into Array(array=w576, new element=w570) -> (w577:string[][])  [unwired: 2 in]
            n218 = call <vilib>:"Space Constant.vi"() -> ("String"=w599:string)
            n219 = Format Into String(w556) -> (resulting string=w621:string)  [unwired: 3 in, 1 out]
            n220 = property class="Arr (严格)"(reference=w585, "Value"=w586) -> ()  [unwired: 1 in, 2 out]
            n221 = property class="Arr (严格)"(reference=w615, "Value"=w614) -> ()  [unwired: 1 in, 2 out]
            n222 = property class="Arr (严格)"(reference=w578, "Value"=w577) -> ()  [unwired: 1 in, 2 out]
            n223 = Concatenate Strings(w599, "水质：" ("字符串"), w621) -> (w622:string)
            n224 = Write to Text File(file (use dialog)=w618, text=w622, error in=w617) -> (refnum out=w562:refnum<file>, error out=w561:errorcluster)  [unwired: 1 in, 1 out]
            n225 = call <vilib>:"Space Constant.vi"() -> ("String"=w565:string)
            n226 = Format Into String(w556) -> (resulting string=w564:string)  [unwired: 3 in, 1 out]
            n227 = Concatenate Strings(w565, "压力：" ("字符串"), w564) -> (w563:string)
            n228 = Write to Text File(file (use dialog)=w562, text=w563, error in=w561) -> (refnum out=w560:refnum<file>, error out=w559:errorcluster)  [unwired: 1 in, 1 out]
            n229 = Write to Text File(file (use dialog)=w560, text="\r\n", error in=w559) -> (refnum out=w625:refnum<file>, error out=w627:errorcluster)  [unwired: 1 in, 1 out]
          }
          frame #4 {
          }
          frame #5 {
            n230 = Multiply(x=w663, y=w666) -> (x*y=w660:dbl)
            n231 = Format Into String(format string="%.2f" ("格式字符串"), w663) -> (resulting string=w662:string)  [unwired: 2 in, 1 out]
            n232 = Format Into String(format string="%.2f" ("格式字符串"), w660) -> (resulting string=w659:string)  [unwired: 2 in, 1 out]
            n233 = Format Into String(format string="%.2f" ("格式字符串"), w666) -> (resulting string=w665:string)  [unwired: 2 in, 1 out]
            n234 = Merge Errors(w672, w673) -> (w671:errorcluster)
            n235 = property class="Arr (严格)"(reference=w656) -> (reference out=w669:refnum<vi>, "Value"=w670:string[][])  [unwired: 1 in, 1 out]
            n236 = Build Array(w657, w665, w662, w659, w654, w655, w653) -> (w658:string[])
            n237 = Insert Into Array(array=w670, new element=w658) -> (w668:string[][])  [unwired: 2 in]
            n238 = property class="Arr (严格)"(reference=w669, "Value"=w668) -> ()  [unwired: 1 in, 2 out]
          }
          frame #6 {
            n239 = call "读取输出状态.vi"("VISA resource name"=w679) -> ("x = y?"=w678:bool)  [unwired: 7 in, 3 out]
            n240 = Select(t="WORK", s=w678, f="IDLE") -> (s? t:f=w675:string)
          }
        }
      }
    }
    "Numeric" <- w443
  }
  n241 = Close File(refnum=w36, error in=w37) -> ()  [unwired: 2 out]
